vi "DFD Plot Freq Response (Frequency Vector).vi"(5 "output option":u16(ring) items=["Auto", "Floating-Point Only", "Fixed-Point Only"], 6 "fs [Hz]":dbl=-1.0 format="%.2f", 7 "frequency vector [Hz]":dbl[](array[numeric]), 8 "error in (no error)":errorcluster, 9 "dB on? (T)":bool=TRUE, 10 "phase view":T7, 11 "filter in":T1={"mSRate_Fs"=1.0, "mSRate_Version"="2.0", "mSRate_Comments"="", "mSRate_OrgCoef"={"type"=enum."Undefined", "gain"=1.0, "coef a (k)"=[], "coef b (v)"=[]}, "mSRate_CurCoef"={"type"=enum."Undefined", "gain"=1.0, "coef a (k)"=[], "coef b (v)"=[]}, "mSRate_Quantized?"=FALSE, "mSRate_QCoef"={"type"=enum."Undefined", "gain"=1.0, "coef a (k)"=[], "coef b (v)"=[]}, "mSRate_QSettings"=[], "mSRate_Order"=0, "mSRate_Scaling"={"mSRate_ScaleByPowerOf2?"=FALSE, "mSRate_ScaleType"=enum."No Norm"}} {"mSRate_QSettings"."source" items=["Coef a/k"=0, "Coef b/v"=7, "Input"=1, "Output"=2, "Multiplicand"=3, "Product"=4, "Sum"=5, "Delay"=6, "Gain"=8]}) -> (0 "error out":errorcluster, 1 "phase response":cluster{"bins":dbl[], "response FXP":dbl[]}[](graph), 2 "magnitude response":cluster{"bins":dbl[], "response FXP":dbl[]}[](graph), 3 "filter out":T1={"mSRate_Fs"=1.0, "mSRate_Version"="2.0", "mSRate_Comments"="", "mSRate_OrgCoef"={"type"=enum."Undefined", "gain"=1.0, "coef a (k)"=[], "coef b (v)"=[]}, "mSRate_CurCoef"={"type"=enum."Undefined", "gain"=1.0, "coef a (k)"=[], "coef b (v)"=[]}, "mSRate_Quantized?"=FALSE, "mSRate_QCoef"={"type"=enum."Undefined", "gain"=1.0, "coef a (k)"=[], "coef b (v)"=[]}, "mSRate_QSettings"=[], "mSRate_Order"=0, "mSRate_Scaling"={"mSRate_ScaleByPowerOf2?"=FALSE, "mSRate_ScaleType"=enum."No Norm"}} {"mSRate_QSettings"."source" items=["Coef a/k"=0, "Coef b/v"=7, "Input"=1, "Output"=2, "Multiplicand"=3, "Product"=4, "Sum"=5, "Delay"=6, "Gain"=8]})   [LabVIEW 2017, in "NI_DigFilterLicensed.lvlib"]
doc: "Plots the frequency responses, including the magnitude and phase responses, of a filter."
uses:
  <vilib>/addons/Digital Filter Design/NI_DigFilterLicensed.lvlib
  <vilib>/addons/Digital Filter Design/_Objects.llb/DFD Filter Obj.ctl
  <vilib>/addons/Digital Filter Design/_Objects.llb/DFD Filter Coef.ctl
  <vilib>/addons/Digital Filter Design/_Objects.llb/DFD Filter Structure Type Selector.ctl
  <vilib>/addons/Digital Filter Design/_Objects.llb/dfd_Internal Quantization Settings.ctl
  <vilib>/addons/Digital Filter Design/_Objects.llb/dfd_Internal Quantization Srcs.ctl
  <vilib>/addons/Digital Filter Design/_Objects.llb/DFD Coef Norm Type.ctl
  <vilib>/addons/Digital Filter Design/_Objects.llb/DFD Phase Setting.ctl
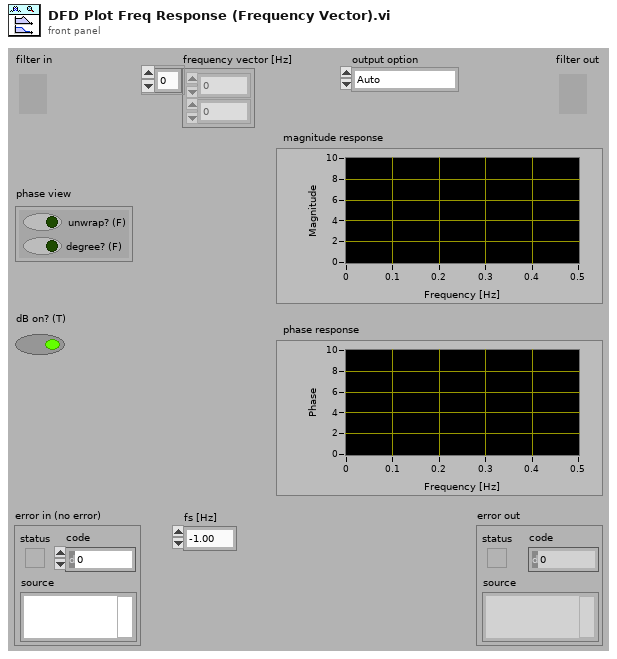
[diagram p1: front panel]
types:
  T1 = typedef "NI_DigFilterLicensed.lvlib/DFD Filter Obj.ctl" = cluster{"mSRate_Fs":dbl, "mSRate_Version":string, "mSRate_Comments":string, "mSRate_OrgCoef":T2, "mSRate_CurCoef":T2, "mSRate_Quantized?":bool, "mSRate_QCoef":T2, "mSRate_QSettings":T4[], "mSRate_Order":i32, "mSRate_Scaling":cluster{"mSRate_ScaleByPowerOf2?":bool, "mSRate_ScaleType":T6}}
  T2 = typedef "NI_DigFilterLicensed.lvlib/DFD Filter Coef.ctl" = cluster{"type":T3, "gain":dbl, "coef a (k)":dbl[], "coef b (v)":dbl[]}
  T3 = typedef "NI_DigFilterLicensed.lvlib/DFD Filter Structure Type Selector.ctl" = enum16{"Undefined", "FIR Direct Form", "FIR Direct Form Transposed", "FIR Symmetric", "FIR Antisymmetric", "IIR Direct Form I", "IIR Direct Form I Transposed", "IIR Direct Form II", "IIR Direct Form II Transposed", "IIR Cascaded Second Order Sections Form I", "IIR Cascaded Second Order Sections Form I Transposed", "IIR Cascaded Second Order Sections Form II", "IIR Cascaded Second Order Sections Form II Transposed", "Lattice Allpass (basic sections)", "Lattice Allpass (one multiplier sections)", "Lattice Allpass (normalized sections)", "Lattice AR (basic sections)", "Lattice AR (one multiplier sections)", "Lattice AR (normalized sections)", "Lattice MA (minimum phase)", "Lattice MA (maximum phase)", "Lattice ARMA (basic sections)", "Lattice ARMA (one multiplier sections)", "Lattice ARMA (normalized sections)"}
  T4 = typedef "NI_DigFilterLicensed.lvlib/dfd_Internal Quantization Settings.ctl" = cluster{"source":T5, "wl":i16, "iwl":i16, "overflow mode":enum16{"Saturation", "Wrap"}, "rounding mode":enum16{"Nearest", "Truncation"}, "signed?":bool}
  T5 = typedef "NI_DigFilterLicensed.lvlib/dfd_Internal Quantization Srcs.ctl" = u16
  T6 = typedef "NI_DigFilterLicensed.lvlib/DFD Coef Norm Type.ctl" = enum16{"No Norm", "Time Domain 1-Norm", "Time Domain 2-Norm", "Time Domain Inf-Norm"}
  T7 = typedef "NI_DigFilterLicensed.lvlib/DFD Phase Setting.ctl" = cluster{"unwrap? (F)":bool, "degree? (F)":bool}
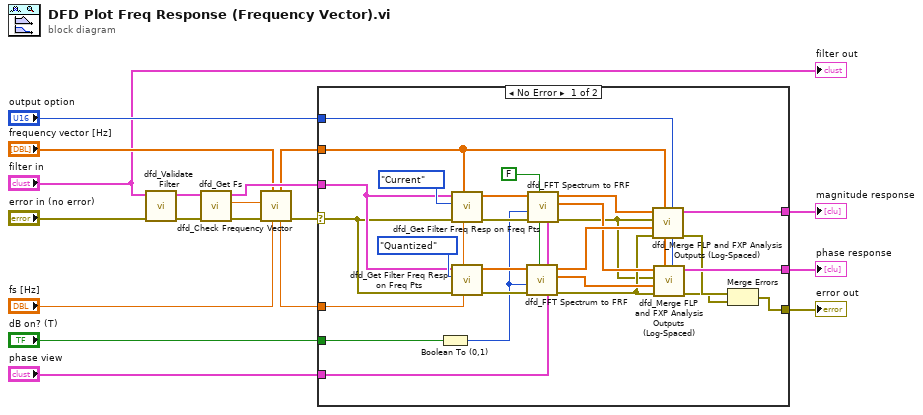
[diagram p0: block diagram]
diagram:
  n1 = call <vilib>:"dfd_Validate Filter.vi"("error in (no error)"="error in (no error)", "filter in"="filter in") -> ("error out"=w12:errorcluster, "filter out"=w13:T1)  [unwired: 1 in, 7 out]
  n2 = call <vilib>:"dfd_Get Fs.vi"("error in (no error)"=w12, "filter in"=w13) -> ("error out"=w10:errorcluster, "fs [Hz]"=w8:dbl, "filter out"=w11:T1)  [unwired: 7 out]
  n3 = call <vilib>:"dfd_Check Frequency Vector.vi"("fs [Hz] in"="fs [Hz]", "frequency vector"="frequency vector [Hz]", "error in (no error)"=w10, "filter fs[Hz]"=w8) -> ("error out"=w9:errorcluster, "fs out [Hz]"=w6:dbl, "frequency vector out"=w4:dbl[])  [unwired: 5 in]
  n4 = case shown="No Error" w9 {
    selector: w9 -> [w21 w45]
    tunnel: "phase view" -> [w33 _]
    tunnel: "dB on? (T)" -> [w42 _]
    tunnel: w6 -> [w23 _]
    tunnel: [w44 w45] -> w16
    tunnel: "output option" -> [w24 _]
    tunnel: [w43 _] -> w2
    tunnel: [w30 _] -> w3
    tunnel: w11 -> [w22 _]
    tunnel: w4 -> [w20 _]
    frame No Error {
      w37 = FALSE ("use half band?")
      n5 = Boolean To (0,1)(Boolean=w42) -> (0, 1=w34:i16)
      n6 = call <vilib>:"dfd_Get Filter Freq Resp on Freq Pts.vi"("fs [Hz]"=w23, "freqs [Hz]"=w20, "error in (no error)"=w21, "coef source"=enum16{"Original", "Current", "Quantized"}."Current", "filter in"=w22) -> ("error out"=w39:errorcluster, "freq response"=w40:cdb[])  [unwired: 3 in, 2 out]
      n7 = call <vilib>:"dfd_Get Filter Freq Resp on Freq Pts.vi"("fs [Hz]"=w23, "freqs [Hz]"=w20, "error in (no error)"=w21, "coef source"=enum16{"Original", "Current", "Quantized"}."Quantized", "filter in"=w22) -> ("error out"=w35:errorcluster, "freq response"=w36:cdb[])  [unwired: 3 in, 2 out]
      n8 = call <vilib>:"dfd_FFT Spectrum to FRF.vi"("phase view"=w33, "use half band?"=w37, "error in (no error)"=w35, "magnitude"=w34, "FFT {X}"=w36) -> ("error out"=w27:errorcluster, "phase"=w28:dbl[], "amplitude"=w31:dbl[])  [unwired: 1 in, 3 out]
      n9 = call <vilib>:"dfd_FFT Spectrum to FRF.vi"("phase view"=w33, "use half band?"=w37, "error in (no error)"=w39, "magnitude"=w34, "FFT {X}"=w40) -> ("error out"=w26:errorcluster, "phase"=w29:dbl[], "amplitude"=w32:dbl[])  [unwired: 1 in, 3 out]
      n10 = call <vilib>:"dfd_Merge FLP and FXP Analysis Outputs (Log-Spaced).vi"("output option"=w24, "frequency points"=w20, "error in FXP"=w27, "response FXP"=w31, "error in FLP"=w26, "response FLP"=w32) -> ("error out"=w25:errorcluster, "freq responses"=w30:cluster{"bins":dbl[], "response FXP":dbl[]}[])  [unwired: 4 in]
      n11 = call <vilib>:"dfd_Merge FLP and FXP Analysis Outputs (Log-Spaced).vi"("output option"=w24, "frequency points"=w20, "error in FXP"=w27, "response FXP"=w28, "error in FLP"=w26, "response FLP"=w29) -> ("error out"=w19:errorcluster, "freq responses"=w43:cluster{"bins":dbl[], "response FXP":dbl[]}[])  [unwired: 4 in]
      n12 = Merge Errors(w25, w19) -> (w44:errorcluster)
    }
    frame Error {
    }
  }
  "error out" <- w16
  "magnitude response" <- w3
  "phase response" <- w2
  "filter out" <- "filter in"
